vi "FRIC_navX_Internal_USB_ProcessingLoop.vi"(7 "Device Number":T3, 10 "Serial Port":T2=enum."USB 1", 11 "Rate (4Hz-200Hz)":u8=50 min=4 max=200) -> ()   [LabVIEW 2016]
doc: "This navX VI handles the reading/writing for the navX. All of the good stuff is in here.\nTHIS VI SHOULD NOT BE CALLED BY THE USER!"
uses:
  _TypeDefs/Z900_navX_SerialStreamTypeDef.ctl
  _TypeDefs/FRIC_navX_DeviceNumbersTypeDef.ctl
  <vilib>/Rock Robotics/WPI/SerialPort/WPI_SerialPort.ctl
  _TypeDefs/FRIC_navX_I2C Process Loop TypeDef.ctl
  _TypeDefs/FRIC_navX_ProcessingLoopStatesTypeDef_I2C.ctl
  _TypeDefs/Z900_navX_DeviceTypeDef.ctl
  _TypeDefs/Z900_navX_ProtocolTypeDef.ctl
  _TypeDefs/Z900_navX_NotifyPacketTypeDef.ctl
  _TypeDefs/Z900_navX_ActionTypeDef.ctl
  <vilib>/Rock Robotics/SystemInterfaces/i2clib/i2c_bus.ctl
  _TypeDefs/Z900_navX_IntegrationControlRegisters.ctl
  <vilib>/Rock Robotics/WPI/SPI/WPI_SPIDevRef.ctl
  <vilib>/Rock Robotics/SystemInterfaces/spilib/spi_bus.ctl
  <vilib>/Rock Robotics/WPI/SerialPort/WPI_SerialPortRef.ctl
  <vilib>/Platform/TimedLoop/XDataNode/timing_clust.ctl
  <vilib>/Platform/TimedLoop/XDataNode/nitl_modes.ctl
  <vilib>/Platform/TimedLoop/XDataNode/wakeup.ctl
  <vilib>/Rock Robotics/SystemInterfaces/Utilities/FPGA_UtilitiesRead LocalTime.vi
  <vilib>/Platform/TimedLoop/XDataNode/XDataNode.xnode
  <vilib>/Platform/TimedLoop/XDataNode/XDNodeRunTimeDep.lvlib
  <vilib>/ptbypt/NI_PtbyPt.lvlib
panel:
  in  "Tab Control":enum32{"Page 1", "Page 2"}(tab)
  in  "Halt":bool
  out "Connected 2":bool
  out "error":errorcluster
  in  "Stream Type":T1=enum."AHRSAndPositioning"
  out "Loop Time":dbl format="%#.1g"
  out "Loop dt":i64
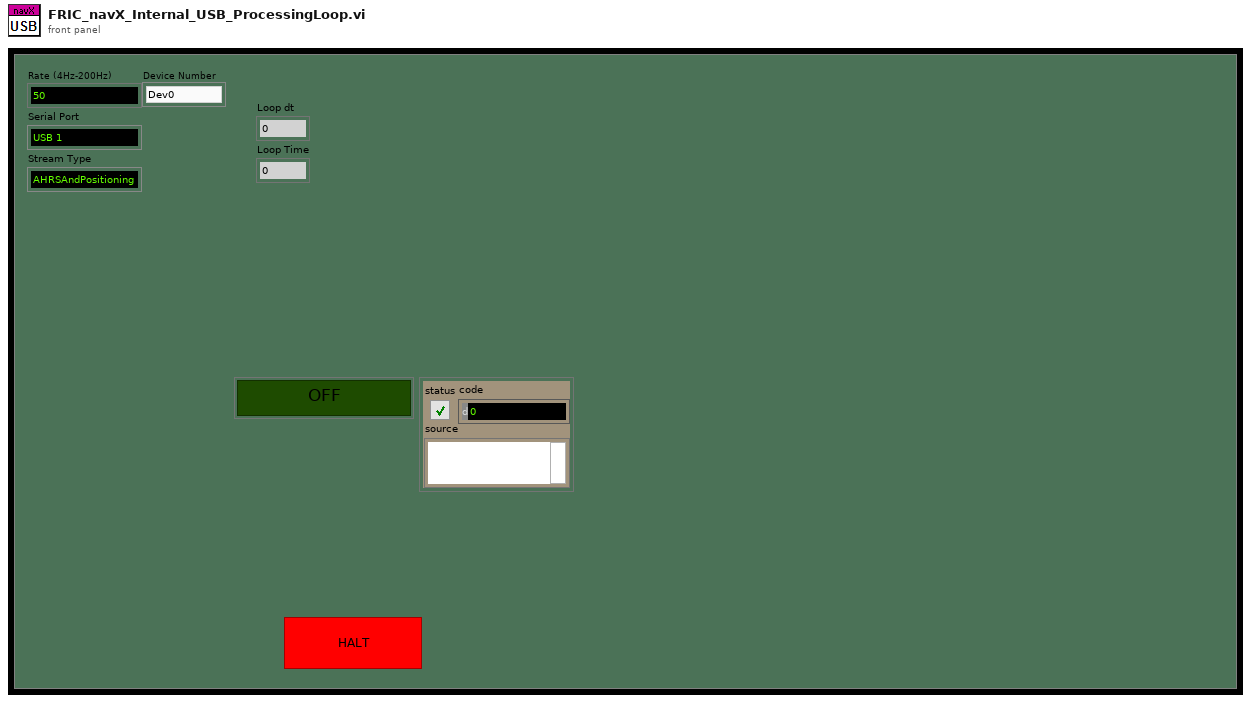
[diagram p1: front panel]
types:
  T1 = typedef "Z900_navX_SerialStreamTypeDef.ctl" = enum16{"YRPH", "Quaterinons", "Gyro/Raw", "AHRS", "AHRSAndPositioning", "AHRSAndPOSTime"}
  T2 = typedef "WPI_SerialPort.ctl" = enum16{"Onboard RS-232", "MXP TTL", "USB 1", "USB 2"}
  T3 = typedef "FRIC_navX_DeviceNumbersTypeDef.ctl" = enum16{"Dev0", "Dev1", "Dev2", "Dev3"}
  T4 = typedef "FRIC_navX_I2C Process Loop TypeDef.ctl" = cluster{"State Array":T5[], "error":errorcluster, "FPGA Cluster":cluster{"Last Valid FPGA Time":dbl, "Error Count":i32, "Initialized":bool}, "Device Info":T6, "I2CDevRef":cluster{"DevStatus":errorcluster, "Device Address":u8, "Handle":i32, "I2C Bus":T8}, "Registry":u8[], "Command Array":T9[], "Connected?":bool, "navX Device Memory Size":i32, "notification":T10, "Memory Size Set":bool, "SPIDevRef":T12, "navX Serial Open":cluster{"Stream Type":T1, "Serial Port":T2}, "SerialPortRef":T14, "Serial Read Buffer":string, "Serial Write Buffer":string[], "Device Number":T3, "navX SPI Open":cluster{"SPI Bus":T13, "Clock Rate (Hz)":dbl}, "Loop dt":i64, "current time":timestamp, "Loop Time":i64}
  T5 = typedef "FRIC_navX_ProcessingLoopStatesTypeDef_I2C.ctl" = enum16{"Process", "INI", "Check Packets Valid", "Close", "Flush Serial", "Generate Command", "Last Packet Valid", "Open", "Read", "Reset Serial", "Set Termination Char", "Update AE", "Wait", "Write", "Exit"}
  T6 = typedef "Z900_navX_DeviceTypeDef.ctl" = cluster{"Interface":cluster{"Protocol":T7, "Update Rate (4Hz-200Hz)":u8, "navX Open TypeDef":variant}, "Notify Packet":refnum<notifier>, "Loop VI Refnum":refnum<vi>, "Ready to Close Occurrence Refnum":refnum<k4>, "Name":string}
  T7 = typedef "Z900_navX_ProtocolTypeDef.ctl" = enum16{"SERIAL", "I2C", "SPI"}
  T8 = typedef "i2c_bus.ctl" = enum16{"I2C On-Board", "I2C MXP", "Invalid"}
  T9 = typedef "Z900_navX_IntegrationControlRegisters.ctl" = u8
  T10 = typedef "Z900_navX_NotifyPacketTypeDef.ctl" = cluster{"navX Action":T11, "Data":variant, "Stream Type":T1, "Device Number":T3}
  T11 = typedef "Z900_navX_ActionTypeDef.ctl" = enum16{"None", "Halt", "Normal Read", "Update Serial Protocol", "Update Rate Htz", "Zero-Yaw", "Zero-Displacement", "Zero-Velocity"}
  T12 = typedef "WPI_SPIDevRef.ctl" = cluster{"DevStatus":errorcluster, "Handle":i32, "SPI Bus":T13}
  T13 = typedef "spi_bus.ctl" = enum16{"SPI On-Board, CS0", "SPI On-Board, CS1", "SPI On-Board, CS2", "SPI On-Board, CS3", "SPI MXP", "Invalid"}
  T14 = typedef "WPI_SerialPortRef.ctl" = cluster{"DevStatus":errorcluster, "Serial Port Name":refnum<visa-resource-name>}
  T15 = typedef "XDNodeRunTimeDep.lvlib/timing_clust.ctl" = cluster{"Expected End [f-1]":u64, "Actual End [f-1]":u64, "Finished Late? [f-1]":bool, "Expected End [i-1]":u64, "Actual End [i-1]":u64, "Finished Late? [i-1]":bool, "Expected Start [i]":u64, "Actual Start [i]":u64, "Expected Start [f]":u64, "Actual Start [f]":u64, "Source Name":string, "Structure Name":string, "Period":i64, "Deadline":i64, "Offset":i64, "Start":i64, "Priority":i32, "Timeout":i32, "Mode":T16, "Wakeup Reason":T17, "Error":errorcluster, "Source Type":string, "Secondary Source Type":string, "Global End Time":u64, "Global Start Time":u64, "Frame Duration":u64, "Iteration Duration":u64, "Assigned CPU":i32, "I/O Scan Engine Mode":u32}
  T16 = typedef "XDNodeRunTimeDep.lvlib/nitl_modes.ctl" = enum32{"No Change", "Process missed periods, maintain original phase", "Discard missed periods, maintain original phase", "Process missed periods, ignore original phase", "Discard missed periods, ignore original phase"}
  T17 = typedef "XDNodeRunTimeDep.lvlib/wakeup.ctl" = enum32{"Normal", "Aborted", "Asynchronous wakeup", "Timing source error", "Timed loop error", "Timeout"}
  T18 = cluster{"Last Valid FPGA Time":dbl, "Error Count":i32, "Initialized":bool}
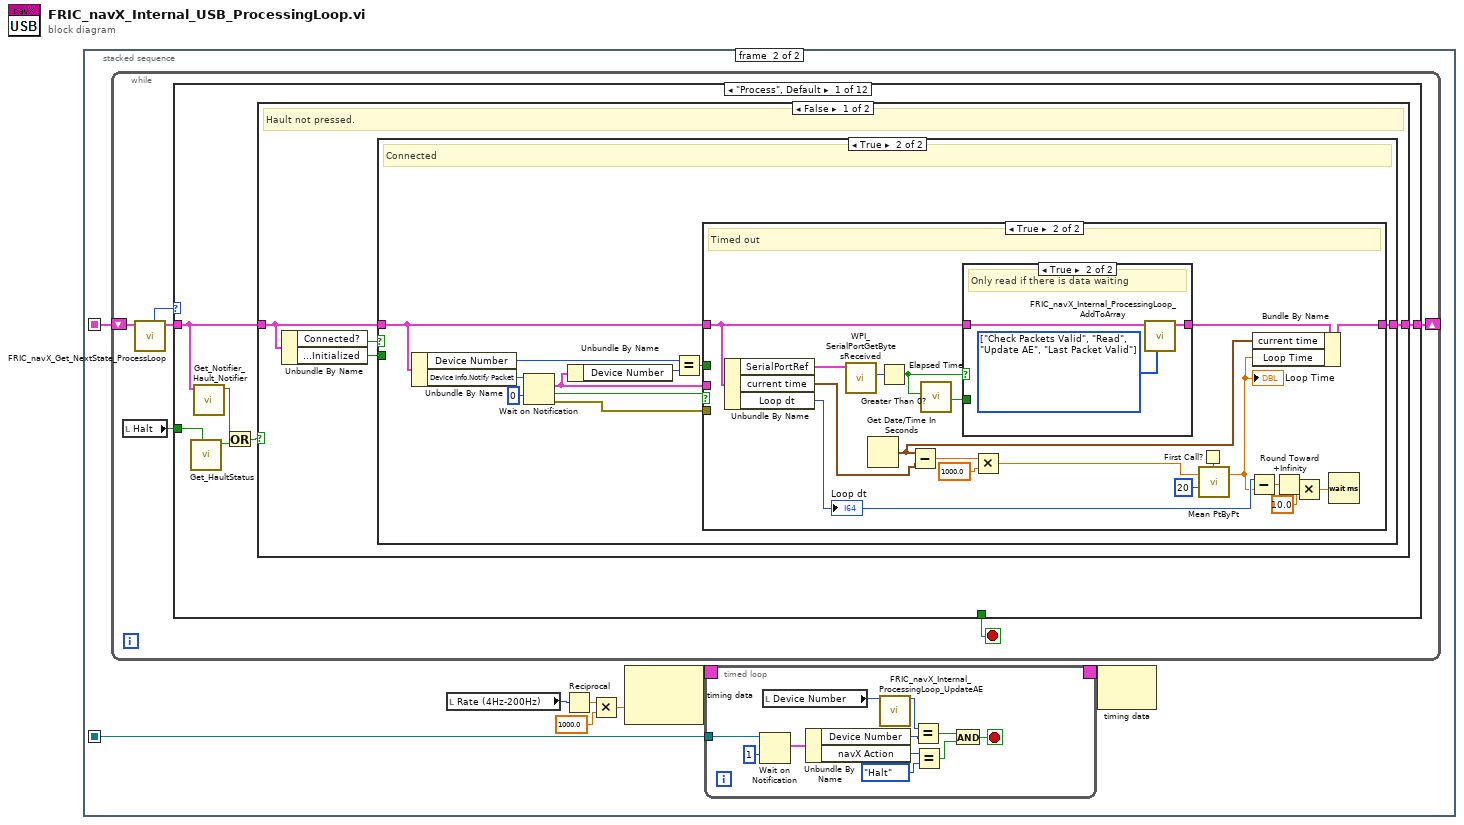
[diagram p0: block diagram]
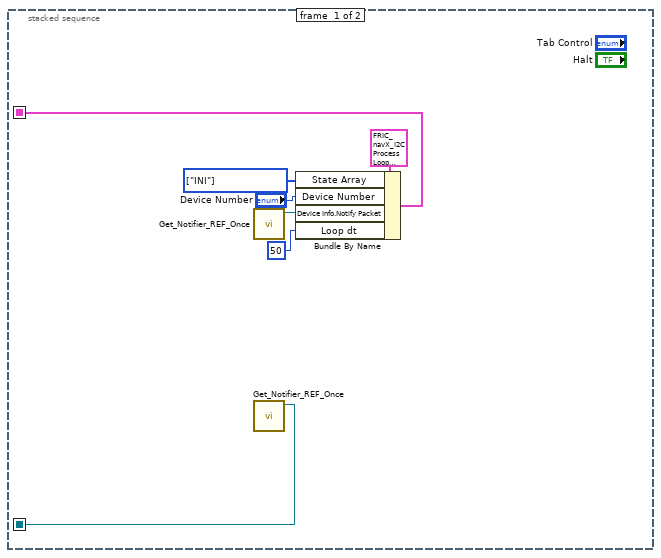
[diagram p2: hidden frame]
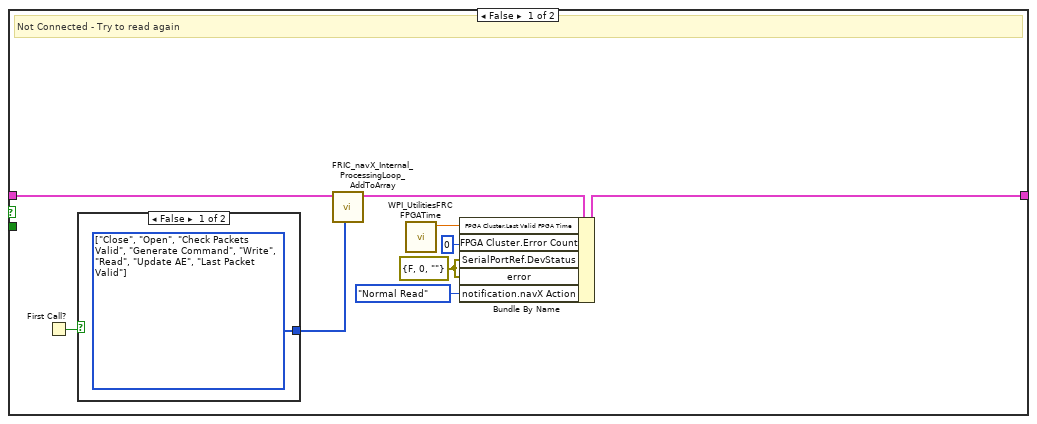
[diagram p3: hidden frame]
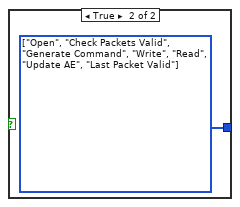
[diagram p4: hidden frame]
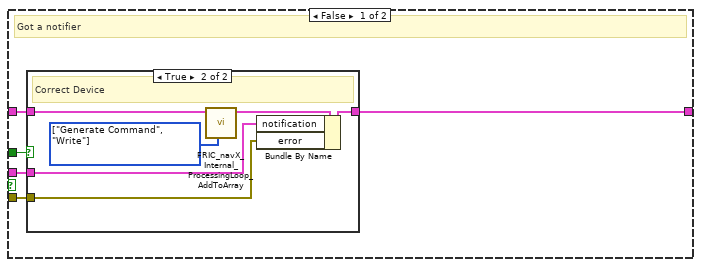
[diagram p5: hidden frame]
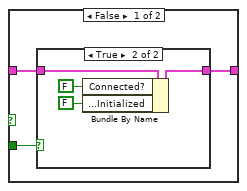
[diagram p7: hidden frame]
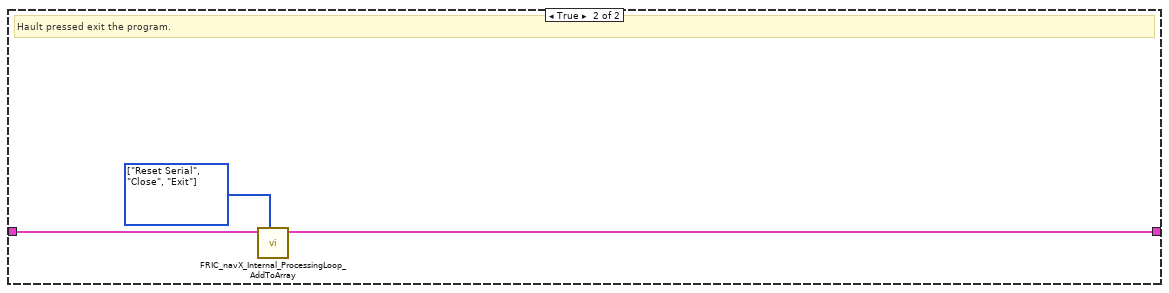
[diagram p9: hidden frame]
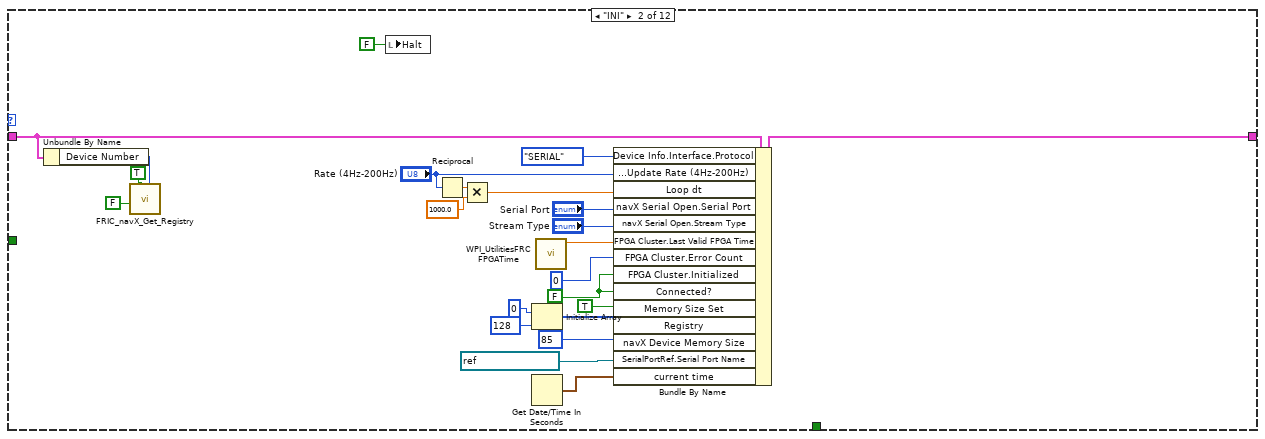
[diagram p10: hidden frame]
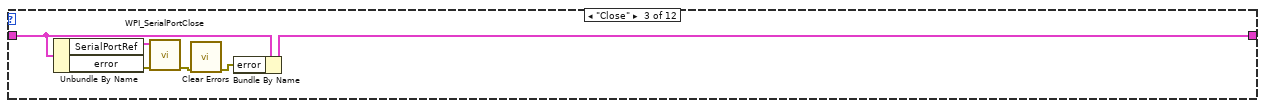
[diagram p11: hidden frame]
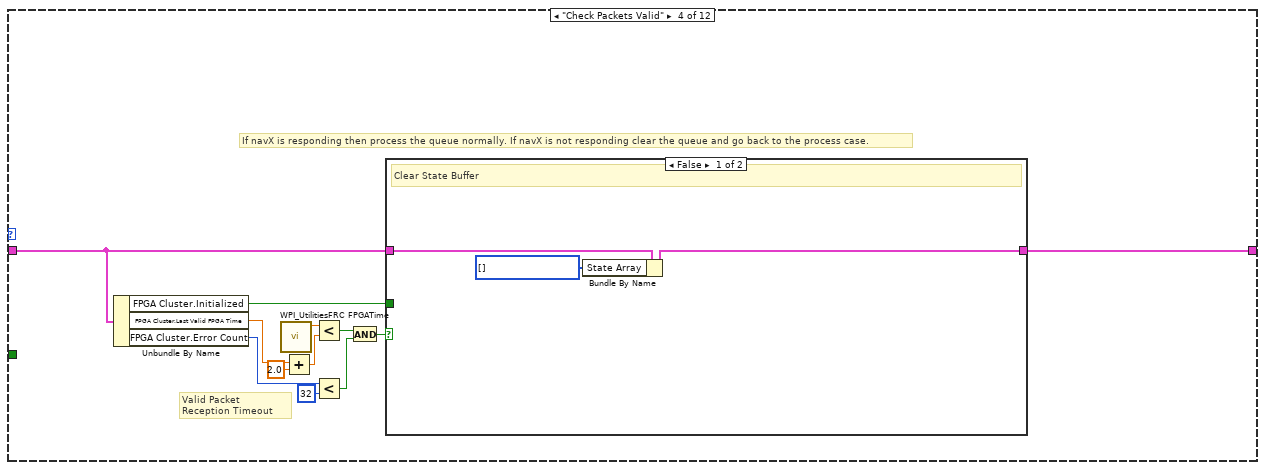
[diagram p12: hidden frame]
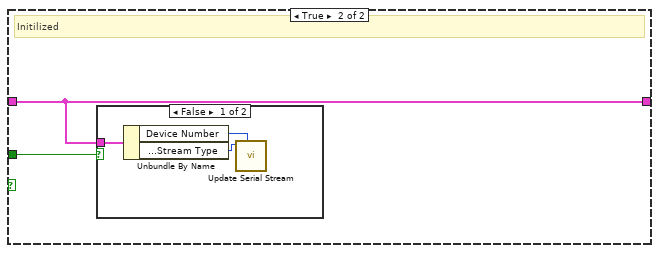
[diagram p13: hidden frame]
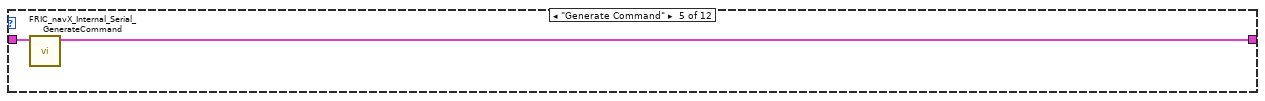
[diagram p15: hidden frame]
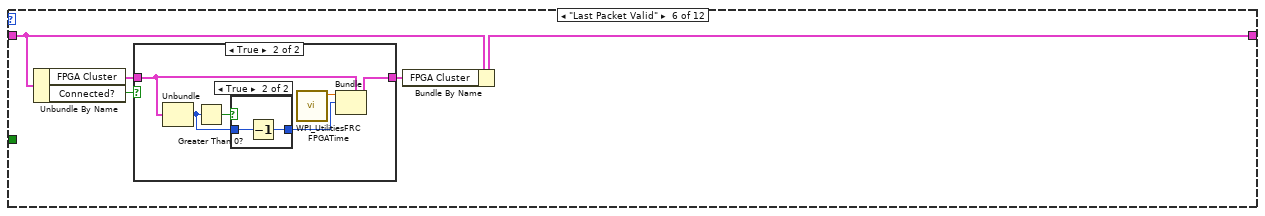
[diagram p16: hidden frame]
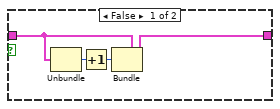
[diagram p17: hidden frame]
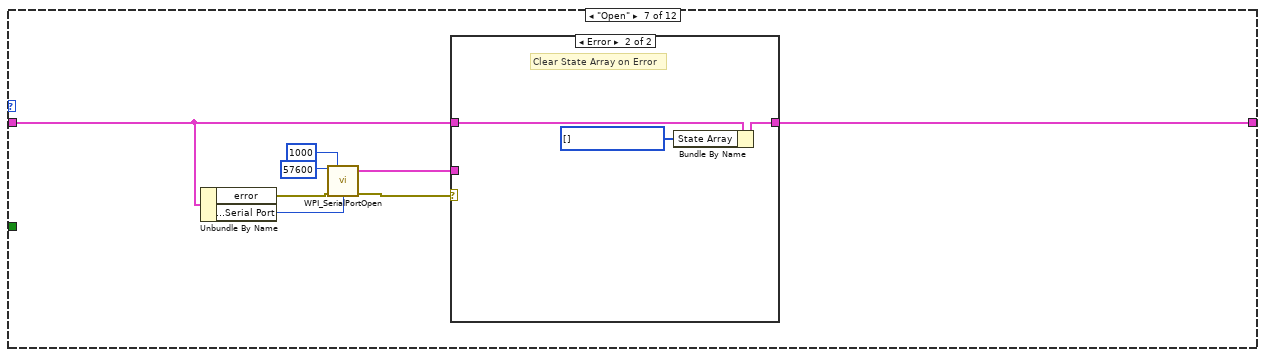
[diagram p19: hidden frame]
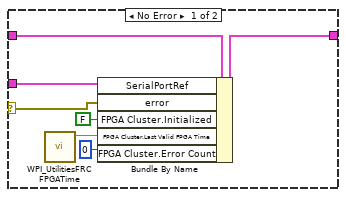
[diagram p20: hidden frame]
diagram:
  n1 = stacked-sequence {
    seq-local: [w7 _] -> [_ w15]
    seq-local: [w1 _] -> [_ w8]
    frame #0 {
      w5 = T5[] [enum."INI"] items=["Process", "INI", "Check Packets Valid", "Close", "Flush Serial", "Generate Command", "Last Packet Valid", "Open", "Read", "Reset Serial", "Set Termination Char", "Update AE", "Wait", "Write", "Exit"] ("State Array")
      n2 = call "Get_Notifier_REF_Once.vi"() -> ("notifier ref out"=w3:refnum<notifier>)  [unwired: 10 in, 1 out]
      n3 = call "Get_Notifier_REF_Once.vi"() -> ("notifier ref out"=w1:refnum<notifier>)  [unwired: 10 in, 1 out]
      n4 = Bundle By Name(cluster=T4 {"State Array"=[enum."INI", enum."Open"], "error"={"status"=FALSE, "code"=0, "source"=""}, "FPGA Cluster"={"Last Valid FPGA Time"=0.0, "Error Count"=0, "Initialized"=FALSE}, "Device Info"={"Interface"={"Protocol"=enum."SERIAL", "Update Rate (4Hz-200Hz)"=4, "navX Open TypeDef"=variant}, "Notify Packet"=refnum, "Loop VI Refnum"=refnum, "Ready to Close Occurrence Refnum"=refnum, "Name"=""}, "I2CDevRef"={"DevStatus"={"status"=FALSE, "code"=0, "source"=""}, "Device Address"=0, "Handle"=0, "I2C Bus"=enum."Invalid"}, "Registry"=[], "Command Array"=[214, 32], "Connected?"=FALSE, "navX Device Memory Size"=85, "notification"={"navX Action"=enum."None", "Data"=variant, "Stream Type"=enum."YRPH", "Device Number"=enum."Dev0"}, "Memory Size Set"=FALSE, "SPIDevRef"={"DevStatus"={"status"=FALSE, "code"=0, "source"=""}, "Handle"=0, "SPI Bus"=enum."SPI On-Board, CS0"}, "navX Serial Open"={"Stream Type"=enum."YRPH", "Serial Port"=enum."Onboard RS-232"}, "SerialPortRef"={"DevStatus"={"status"=FALSE, "code"=0, "source"=""}, "Serial Port Name"=""}, "Serial Read Buffer"="", "Serial Write Buffer"=[], "Device Number"=enum."Dev0", "navX SPI Open"={"SPI Bus"=enum."SPI MXP", "Clock Rate (Hz)"=500000.0}, "Loop dt"=0, "current time"=timestamp(0 s since 1904-01-01), "Loop Time"=0} ("I2C Process Loop TypeDef"), "State Array"=w5, "Device Number"="Device Number", "Device Info.Notify Packet"=w3, "Loop dt"=i64 50) -> (w7:T4)
    }
    frame #1 {
      n5 = while {
        shift-right: [w33] -> _
        shift-left: w15 -> [w36]
        stop <- w37 stop-if-true
        n6 = local read "Halt"() -> (w32:bool)
        n7 = call "FRIC_navX_Get_NextState_ProcessLoop.vi"("I2C Process Loop TypeDef (in)"=w36) -> ("I2C Process Loop TypeDef (out)"=w35:T4, "Current State"=w34:T5)  [unwired: 9 in]
        n8 = case shown="\"Process\", Default" w34 {
          tunnel: [_ _ _ _ _ _ _ _ _ _ TRUE _] -> w37
          tunnel: w35 -> [w41 w125 w143 w148 w165 w169 w191 w219 w237 w250 w257 w265]
          tunnel: [w43 w132 w142 w149 w164 w168 w190 w211 w238 w239 w257 w265] -> w33
          tunnel: w32 -> [w42 _ _ _ _ _ _ _ _ _ _ _]
          frame "Process", Default {
            n9 = call "Get_HaultStatus.vi"("Update"=w42) -> ("Hault"=w39:bool)  [unwired: 10 in]
            n10 = call "Get_Notifier_Hault_Notifier.vi"("Process Loop TypeDef (in)"=w41) -> ("Hault Notifier"=w40:bool)  [unwired: 10 in]
            n11 = Or(x=w40, y=w39) -> (x .or. y?=w38:bool)
            n12 = case shown="False" w38 {
              tunnel: [w47 w113] -> w43
              tunnel: w41 -> [w45 w114]
              frame False {
                # "Hault not pressed."
                n13 = Unbundle By Name(w45) -> ("Connected?"=w46:bool, "FPGA Cluster.Initialized"=w44:bool)
                n14 = case shown="True" w46 {
                  tunnel: w45 -> [w56 w59]
                  tunnel: [w53 w68] -> w47
                  tunnel: w44 -> [_ _]
                  frame False {
                    w50 = errorcluster {"status"=FALSE, "code"=0, "source"=""} ("SerialPortRef.DevStatus")
                    # "Not Connected - Try to read again"
                    n15 = First Call?() -> (First Call?: T/F=w49:bool)
                    n16 = case shown="False" w49 {
                      tunnel: [w57 w58] -> w55
                      frame False {
                        w57 = T5[] [enum."Close", enum."Open", enum."Check Packets Valid", enum."Generate Command", enum."Write", enum."Read", enum."Update AE", enum."Last Packet Valid"] items=["Process", "INI", "Check Packets Valid", "Close", "Flush Serial", "Generate Command", "Last Packet Valid", "Open", "Read", "Reset Serial", "Set Termination Char", "Update AE", "Wait", "Write", "Exit"]
                      }
                      frame True {
                        w58 = T5[] [enum."Open", enum."Check Packets Valid", enum."Generate Command", enum."Write", enum."Read", enum."Update AE", enum."Last Packet Valid"] items=["Process", "INI", "Check Packets Valid", "Close", "Flush Serial", "Generate Command", "Last Packet Valid", "Open", "Read", "Reset Serial", "Set Termination Char", "Update AE", "Wait", "Write", "Exit"]
                      }
                    }
                    n17 = call "FRIC_navX_Internal_ProcessingLoop_AddToArray.vi"("States Array"=w55, "I2C Process Loop TypeDef (in)"=w56) -> ("I2C Process Loop TypeDef (out)"=w54:T4)  [unwired: 9 in]
                    n18 = call <vilib>:"WPI_UtilitiesFRC FPGATime.vi"() -> ("FPGA Time"=w51:dbl)  [unwired: 10 in, 1 out]
                    n19 = Bundle By Name(cluster=w54, "FPGA Cluster.Last Valid FPGA Time"=w51, "FPGA Cluster.Error Count"=0, "SerialPortRef.DevStatus"=w50, "error"=w50, "notification.navX Action"=Z900_navX_ActionTypeDef."Normal Read") -> (w53:T4)
                  }
                  frame True {
                    # "Connected"
                    n20 = Unbundle By Name(w59) -> ("Device Number"=w62:T3, "Device Info.Notify Packet"=w67:refnum<notifier>)
                    n21 = Wait on Notification(notifier=w67, timeout in ms (-1)=0) -> (notification=w63:T10, timed out?=w64:bool, error out=w65:errorcluster)  [unwired: 2 in, 1 out]
                    n22 = Unbundle By Name(w63) -> ("Device Number"=w61:T3)
                    n23 = Equal?(x=w62, y=w61) -> (x = y?=w60:bool)
                    n24 = case shown="True" w64 {
                      tunnel: w59 -> [w73 w97]
                      tunnel: [w72 w94] -> w68
                      tunnel: w63 -> [w71 _]
                      tunnel: w65 -> [w70 _]
                      tunnel: w60 -> [w69 _]
                      frame False {
                        # "Got a notifier"
                        n25 = case shown="True" w69 {
                          tunnel: w73 -> [w74 w80]
                          tunnel: [w74 w79] -> w72
                          tunnel: w71 -> [_ w78]
                          tunnel: w70 -> [_ w75]
                          frame False {
                          }
                          frame True {
                            w76 = T5[] [enum."Generate Command", enum."Write"] items=["Process", "INI", "Check Packets Valid", "Close", "Flush Serial", "Generate Command", "Last Packet Valid", "Open", "Read", "Reset Serial", "Set Termination Char", "Update AE", "Wait", "Write", "Exit"] ("States Array")
                            # "Correct Device"
                            n26 = call "FRIC_navX_Internal_ProcessingLoop_AddToArray.vi"("States Array"=w76, "I2C Process Loop TypeDef (in)"=w80) -> ("I2C Process Loop TypeDef (out)"=w77:T4)  [unwired: 9 in]
                            n27 = Bundle By Name(cluster=w77, "notification"=w78, "error"=w75) -> (w79:T4)
                          }
                        }
                      }
                      frame True {
                        # "Timed out"
                        n28 = Unbundle By Name(w97) -> ("SerialPortRef"=w99:T14, "current time"=w93:timestamp, "Loop dt"=w82:i64)
                        "Loop dt" <- w82
                        n29 = call <vilib>:"WPI_SerialPortGetBytesReceived.vi"("SerialPortRef"=w99) -> ("Bytes at Port"=w98:u32)  [unwired: 8 in, 2 out]
                        n30 = Get Date/Time In Seconds() -> (seconds since 1Jan1904=w92:timestamp)
                        n31 = Greater Than 0?(x=w98) -> (x > 0?=w96:bool)
                        n32 = Subtract(x=w92, y=w93) -> (x-y=w91:dbl)
                        n33 = call "Elapsed Time"("Reset"=w96) -> ("Time has Elapsed"=w95:bool)  [unwired: 11 in, 7 out]
                        n34 = case shown="True" w96 {
                          tunnel: [w102 w110] -> w100
                          tunnel: w97 -> [w103 w109]
                          tunnel: w95 -> [w101 _]
                          frame False {
                            n35 = case shown="True" w101 {
                              tunnel: w103 -> [w104 w108]
                              tunnel: [w104 w107] -> w102
                              frame False {
                              }
                              frame True {
                                n36 = Bundle By Name(cluster=w108, "Connected?"=FALSE, "FPGA Cluster.Initialized"=FALSE) -> (w107:T4)
                              }
                            }
                          }
                          frame True {
                            w111 = T5[] [enum."Check Packets Valid", enum."Read", enum."Update AE", enum."Last Packet Valid"] items=["Process", "INI", "Check Packets Valid", "Close", "Flush Serial", "Generate Command", "Last Packet Valid", "Open", "Read", "Reset Serial", "Set Termination Char", "Update AE", "Wait", "Write", "Exit"]
                            # "Only read if there is data waiting"
                            n37 = call "FRIC_navX_Internal_ProcessingLoop_AddToArray.vi"("States Array"=w111, "I2C Process Loop TypeDef (in)"=w109) -> ("I2C Process Loop TypeDef (out)"=w110:T4)  [unwired: 9 in]
                          }
                        }
                        n38 = Multiply(x=w91, y=1000.0) -> (x*y=w83:dbl)
                        n39 = First Call?() -> (First Call?: T/F=w85:bool)
                        n40 = call <vilib>:"Mean PtByPt.vi"("x"=w83, "sample length"=20, "initialize"=w85) -> ("mean"=w81:dbl)  [unwired: 1 in, 1 out]
                        "Loop Time" <- w81
                        n41 = Subtract(x=w82, y=w81) -> (x-y=w87:dbl)
                        n42 = Bundle By Name(cluster=w100, "current time"=w92, "Loop Time"=w81) -> (w94:T4)
                        n43 = Round Toward +Infinity(x=w87) -> (ceil(x): smallest int >= x=w89:dbl)
                        n44 = Multiply(x=w89, y=10.0) -> (x*y=w84:dbl)
                        n45 = Wait (ms)(milliseconds to wait=w84) -> ()  [unwired: 1 out]
                      }
                    }
                  }
                }
              }
              frame True {
                w112 = T5[] [enum."Reset Serial", enum."Close", enum."Exit"] items=["Process", "INI", "Check Packets Valid", "Close", "Flush Serial", "Generate Command", "Last Packet Valid", "Open", "Read", "Reset Serial", "Set Termination Char", "Update AE", "Wait", "Write", "Exit"] ("States Array")
                # "Hault pressed exit the program."
                n46 = call "FRIC_navX_Internal_ProcessingLoop_AddToArray.vi"("States Array"=w112, "I2C Process Loop TypeDef (in)"=w114) -> ("I2C Process Loop TypeDef (out)"=w113:T4)  [unwired: 9 in]
              }
            }
          }
          frame "INI" {
            w130 = FALSE ("Initialized")
            n47 = Unbundle By Name(w125) -> ("Device Number"=w124:T3)
            n48 = call "FRIC_navX_Get_Registry.vi"("Device Number"=w124, "Update"=TRUE, "Connected?"=FALSE) -> ()  [unwired: 7 in, 2 out]
            n49 = local write "Halt"(FALSE ("Halt")) -> ()
            n50 = Reciprocal(x="Rate (4Hz-200Hz)") -> (1/x=w118:dbl)
            n51 = Multiply(x=w118, y=1000.0) -> (x*y=w116:dbl)
            n52 = Initialize Array(u8 0 ("Received Data"), 128 ("hex")) -> (w128:u8[])
            n53 = Get Date/Time In Seconds() -> (seconds since 1Jan1904=w115:timestamp)
            n54 = call <vilib>:"WPI_UtilitiesFRC FPGATime.vi"() -> ("FPGA Time"=w134:dbl)  [unwired: 10 in, 1 out]
            n55 = Bundle By Name(cluster=w125, "Device Info.Interface.Protocol"=Z900_navX_ProtocolTypeDef."SERIAL" ("Protocol"), "Device Info.Interface.Update Rate (4Hz-200Hz)"="Rate (4Hz-200Hz)", "Loop dt"=w116, "navX Serial Open.Serial Port"="Serial Port", "navX Serial Open.Stream Type"="Stream Type", "FPGA Cluster.Last Valid FPGA Time"=w134, "FPGA Cluster.Error Count"=0 ("Error Count"), "FPGA Cluster.Initialized"=w130, "Connected?"=w130, "Memory Size Set"=TRUE, "Registry"=w128, "navX Device Memory Size"=85 ("hex"), "SerialPortRef.Serial Port Name"=refnum<visa-resource-name> "ASRL3::INSTR" ("Serial Port Name"), "current time"=w115) -> (w132:T4)
          }
          frame "Close" {
            n56 = Unbundle By Name(w143) -> ("SerialPortRef"=w140:T14, "error"=w139:errorcluster)
            n57 = call <vilib>:"WPI_SerialPortClose.vi"("error in (no error)"=w139, "SerialPortRef"=w140) -> ("error out"=w138:errorcluster)  [unwired: 9 in]
            n58 = call <vilib>:"Clear Errors.vi"("error in (no error)"=w138) -> ("error out"=w141:errorcluster)  [unwired: 5 in, 1 out]
            n59 = Bundle By Name(cluster=w143, "error"=w141) -> (w142:T4)
          }
          frame "Check Packets Valid" {
            # "If navX is responding then process the queue normally. If navX is not responding clear the queue and go back to the process case."
            # "Valid Packet Reception Timeout"
            n60 = Unbundle By Name(w148) -> ("FPGA Cluster.Initialized"=w144:bool, "FPGA Cluster.Last Valid FPGA Time"=w147:dbl, "FPGA Cluster.Error Count"=w146:i32)
            n61 = call <vilib>:"WPI_UtilitiesFRC FPGATime.vi"() -> ("FPGA Time"=w153:dbl)  [unwired: 10 in, 1 out]
            n62 = Add(x=w147, y=2.0) -> (x+y=w154:dbl)
            n63 = Less?(x=w153, y=w154) -> (x < y?=w151:bool)
            n64 = Less?(x=w146, y=32) -> (x < y?=w150:bool)
            n65 = And(x=w151, y=w150) -> (x .and. y?=w145:bool)
            n66 = case shown="False" w145 {
              tunnel: w148 -> [w158 w160]
              tunnel: [w157 w160] -> w149
              tunnel: w144 -> [_ w159]
              frame False {
                w156 = T5[] [] items=["Process", "INI", "Check Packets Valid", "Close", "Flush Serial", "Generate Command", "Last Packet Valid", "Open", "Read", "Reset Serial", "Set Termination Char", "Update AE", "Wait", "Write", "Exit"] ("f")
                # "Clear State Buffer"
                n67 = Bundle By Name(cluster=w158, "State Array"=w156) -> (w157:T4)
              }
              frame True {
                # "Initilized"
                n68 = case shown="False" w159 {
                  tunnel: w160 -> [w161 _]
                  frame False {
                    n69 = Unbundle By Name(w161) -> ("Device Number"=w162:T3, "navX Serial Open.Stream Type"=w163:T1)
                    n70 = call "Update Serial Stream.vi"("Device Number"=w162, "Stream Type"=w163) -> ()  [unwired: 10 in]
                  }
                  frame True {
                  }
                }
              }
            }
          }
          frame "Generate Command" {
            n71 = call "FRIC_navX_Internal_Serial_GenerateCommand.vi"("Serial Process Loop TypeDef (in)"=w165) -> ("Serial Process Loop TypeDef (out)"=w164:T4)  [unwired: 10 in]
          }
          frame "Last Packet Valid" {
            n72 = Unbundle By Name(w169) -> ("FPGA Cluster"=w170:T18, "Connected?"=w166:bool)
            n73 = case shown="True" w166 {
              tunnel: [w173 w180] -> w167
              tunnel: w170 -> [w172 w176]
              frame False {
                n74 = Unbundle(w172) -> ("Error Count"=w171:i32)  [unwired: 2 out]
                n75 = Increment(x=w171) -> (x+1=w174:i32)
                n76 = Bundle(cluster=w172, "Error Count"=w174) -> (w173:T18)  [unwired: 2 in]
              }
              frame True {
                n77 = Unbundle(w176) -> ("Error Count"=w175:i32)  [unwired: 2 out]
                n78 = Greater Than 0?(x=w175) -> (x > 0?=w178:bool)
                n79 = case shown="True" w178 {
                  tunnel: [w181 w183] -> w177
                  tunnel: w175 -> [w181 w182]
                  frame False {
                  }
                  frame True {
                    n80 = Decrement(x=w182) -> (x-1=w183:i32)
                  }
                }
                n81 = call <vilib>:"WPI_UtilitiesFRC FPGATime.vi"() -> ("FPGA Time"=w179:dbl)  [unwired: 10 in, 1 out]
                n82 = Bundle(cluster=w176, "Last Valid FPGA Time"=w179, "Error Count"=w177) -> (w180:T18)  [unwired: 1 in]
              }
            }
            n83 = Bundle By Name(cluster=w169, "FPGA Cluster"=w167) -> (w168:T4)
          }
          frame "Open" {
            n84 = Unbundle By Name(w191) -> ("error"=w187:errorcluster, "navX Serial Open.Serial Port"=w184:T2)
            n85 = call <vilib>:"WPI_SerialPortOpen.vi"("Baud Rate"=u32 57600, "Timeout Value (ms)"=u32 1000, "error in (no error)"=w187, "Serial Port"=w184) -> ("SerialPortRef"=w189:T14, "error out"=w188:errorcluster)  [unwired: 10 in]
            n86 = case shown="Error" w188 {
              selector: w188 -> [w192 _]
              tunnel: w191 -> [w198 w201]
              tunnel: [w197 w200] -> w190
              tunnel: w189 -> [w195 _]
              frame No Error {
                n87 = call <vilib>:"WPI_UtilitiesFRC FPGATime.vi"() -> ("FPGA Time"=w194:dbl)  [unwired: 10 in, 1 out]
                n88 = Bundle By Name(cluster=w198, "SerialPortRef"=w195, "error"=w192, "FPGA Cluster.Initialized"=FALSE ("Initialized"), "FPGA Cluster.Last Valid FPGA Time"=w194, "FPGA Cluster.Error Count"=0) -> (w197:T4)
              }
              frame Error {
                w199 = T5[] [] items=["Process", "INI", "Check Packets Valid", "Close", "Flush Serial", "Generate Command", "Last Packet Valid", "Open", "Read", "Reset Serial", "Set Termination Char", "Update AE", "Wait", "Write", "Exit"] ("State Array")
                # "Clear State Array on Error"
                n89 = Bundle By Name(cluster=w201, "State Array"=w199) -> (w200:T4)
              }
            }
          }
          frame "Read" {
            n90 = Unbundle By Name(w219) -> ("Serial Read Buffer"=w224:string, "SerialPortRef"=w225:T14, "SerialPortRef.Serial Port Name"=w227:refnum<visa-resource-name>, "error"=w226:errorcluster, "Device Number"=w204:T3, "Registry"=w220:u8[])
            n91 = property class="Instr"(reference=w227, error in=w226) -> (error out=w221:errorcluster, "Bytes at Port"=w208:u32)  [unwired: 1 in]
            n92 = Greater?(x=w208, y=u32 512) -> (0:w210:bool)
            n93 = Select(t=u32 512 ("y"), s=w210, f=w208) -> (s? t:f=w207:u32)
            n94 = call <vilib>:"WPI_SerialPortRead.vi"("error in (no error)"=w221, "Num Bytes to Read"=w207, "SerialPortRef"=w225) -> ("error out"=w203:errorcluster, "Buffer"=w218:string)  [unwired: 6 in, 1 out]
            n95 = call "FRIC_navX_Clear_Buffer_Warning.vi"("error in"=w203) -> ("error out"=w202:errorcluster)  [unwired: 10 in]
            n96 = Concatenate Strings(w224, w218) -> (w217:string)
            n97 = Not(x=w202) -> (.not. x?=w209:bool)
            "Connected 2" <- w209
            n98 = call "Z900_navX_SERIAL_CapturePacket.vi"("Buffer"=w217) -> ("Packet"=w214:string, "Buffer"=w216:string)  [unwired: 7 in, 2 out]
            n99 = call "Z900_navX_SERIAL_DecodePacket.vi"("Data (in)"=w220, "Packet (in)"=w214) -> ("empty?"=w206:bool, "Data"=w215:u8[])  [unwired: 6 in, 2 out]
            n100 = Not(x=w206) -> (.not. x?=w205:bool)
            n101 = call "FRIC_navX_Get_Registry.vi"("Device Number"=w204, "Update"=w205, "Connected?"=w209, "Registry (in)"=w215) -> ()  [unwired: 6 in, 2 out]
            n102 = Bundle By Name(cluster=w219, "Serial Read Buffer"=w216, "Connected?"=w209, "error"=w202) -> (w212:T4)
            n103 = call "Get_Connect_Status.vi"("Device Number"=w204, "Update"=TRUE, "Connected"=w209) -> ()  [unwired: 8 in, 1 out]
            n104 = case shown="False" w210 {
              tunnel: w212 -> [w228 w232]
              tunnel: [w228 w231] -> w211
              frame False {
              }
              frame True {
                w230 = T5[] [enum."Read"] items=["Process", "INI", "Check Packets Valid", "Close", "Flush Serial", "Generate Command", "Last Packet Valid", "Open", "Read", "Reset Serial", "Set Termination Char", "Update AE", "Wait", "Write", "Exit"] ("States Array")
                n105 = call "FRIC_navX_Internal_ProcessingLoop_AddToArray.vi"("Add to beginning"=TRUE, "States Array"=w230, "I2C Process Loop TypeDef (in)"=w232) -> ("I2C Process Loop TypeDef (out)"=w231:T4)  [unwired: 8 in]
              }
            }
          }
          frame "Reset Serial" {
            n106 = Unbundle By Name(w237) -> ("SerialPortRef"=w236:T14, "error"=w234:errorcluster)
            n107 = call <vilib>:"WPI_SerialPortReset.vi"("error in (no error)"=w234, "SerialPortRef"=w236) -> ("error out"=w233:errorcluster, "SerialPortRef"=w235:T14)  [unwired: 8 in]
            n108 = Bundle By Name(cluster=w237, "SerialPortRef"=w235, "error"=w233) -> (w238:T4)
          }
          frame "Write" {
            n109 = Unbundle By Name(w250) -> ("SerialPortRef"=w248:T14, "Serial Write Buffer"=w245:string[], "SerialPortRef.DevStatus"=w249:errorcluster)
            n110 = Delete From Array(array=w245, index=0) -> (deleted portion=w244:string, array with subset deleted=w241:string[])  [unwired: 1 in]
            n111 = call <vilib>:"WPI_SerialPortWrite.vi"("error in (no error)"=w249, "Buffer"=w244, "SerialPortRef"=w248) -> ("error out"=w247:errorcluster, "SerialPortRef"=w246:T14)  [unwired: 6 in, 1 out]
            n112 = Empty Array?(array=w241) -> (empty?=w240:bool)
            n113 = Bundle By Name(cluster=w250, "SerialPortRef"=w246, "error"=w247, "Serial Write Buffer"=w241) -> (w242:T4)
            n114 = case shown="False" w240 {
              tunnel: [w254 w255] -> w239
              tunnel: w242 -> [w253 w255]
              frame False {
                w252 = T5[] [enum."Write"] items=["Process", "INI", "Check Packets Valid", "Close", "Flush Serial", "Generate Command", "Last Packet Valid", "Open", "Read", "Reset Serial", "Set Termination Char", "Update AE", "Wait", "Write", "Exit"] ("States Array")
                # "Write again because buffer is not empty."
                n115 = call "FRIC_navX_Internal_ProcessingLoop_AddToArray.vi"("Add to beginning"=TRUE, "States Array"=w252, "I2C Process Loop TypeDef (in)"=w253) -> ("I2C Process Loop TypeDef (out)"=w254:T4)  [unwired: 8 in]
              }
              frame True {
                # "Process the rest of the state array"
              }
            }
          }
          frame "Exit" {
            n116 = Unbundle By Name(w257) -> ("Device Info"=w256:T6)
            n117 = in-place {
              in-place-border: w256 -> [w260]
              # "Set Occurence of Close"
              n118 = Unbundle By Name(w260) -> ("Ready to Close Occurrence Refnum"=w261:refnum<k4>)
              n119 = local write "Halt"(FALSE ("Halt")) -> ()
              n120 = Set Occurrence(w261) -> ()
            }
          }
          frame "Update AE" {
            n121 = Unbundle By Name(w265) -> ("Device Number"=w262:T3, "error"=w264:errorcluster)
            "error" <- w264
            n122 = call "Get_Error_Status.vi"("Device Number"=w262, "Update"=TRUE, "error in"=w264) -> ()  [unwired: 8 in, 1 out]
          }
        }
      }
      n123 = local read "Rate (4Hz-200Hz)"() -> (w13:u8)
      n124 = Reciprocal(x=w13) -> (1/x=w14:dbl)
      n125 = Multiply(x=w14, y=1000.0) -> (x*y=w9:dbl)
      n126 = node-c288(w9) -> (w11:T15)  [unwired: 1 in]
      n127 = timed-loop {
        timing: w11 -> [_]
        timing-out: [_] -> w10
        tunnel: w8 -> [w22]
        stop <- w16 stop-if-true
        n128 = Wait on Notification(notifier=w22, timeout in ms (-1)=1) -> (notification=w21:T10)  [unwired: 2 in, 3 out]
        n129 = local read "Device Number"() -> (w19:T3)
        n130 = Unbundle By Name(w21) -> ("Device Number"=w20:T3, "navX Action"=w24:T11)
        n131 = call "FRIC_navX_Internal_ProcessingLoop_UpdateAE.vi"("Device Number"=w19) -> ()  [unwired: 15 in]
        n132 = Equal?(x=w19, y=w20) -> (x = y?=w18:bool)
        n133 = Equal?(x=w24, y=Z900_navX_ActionTypeDef."Halt") -> (x = y?=w17:bool)
        n134 = And(x=w18, y=w17) -> (x .and. y?=w16:bool)
      }
      n135 = node-c288(w10) -> ()  [unwired: 1 out]
    }
  }
